vi "apply control changes.vi"(9 "new":string[][](array[string]), 10 "old":string[][](array[string]), 11 "Data In":T1[](array[typedef])) -> (1 "Changed indices":i32[](array[numeric]), 3 "Data Out":T1[](array[typedef]))   [LabVIEW 2016, in "update vi properties.lvlib"]
uses:
  update vi properties.lvlib
  Cluster_Data.ctl
  <vilib>/picture/picture.llb/imagedata.ctl
panel:
  # "Connector Pane"
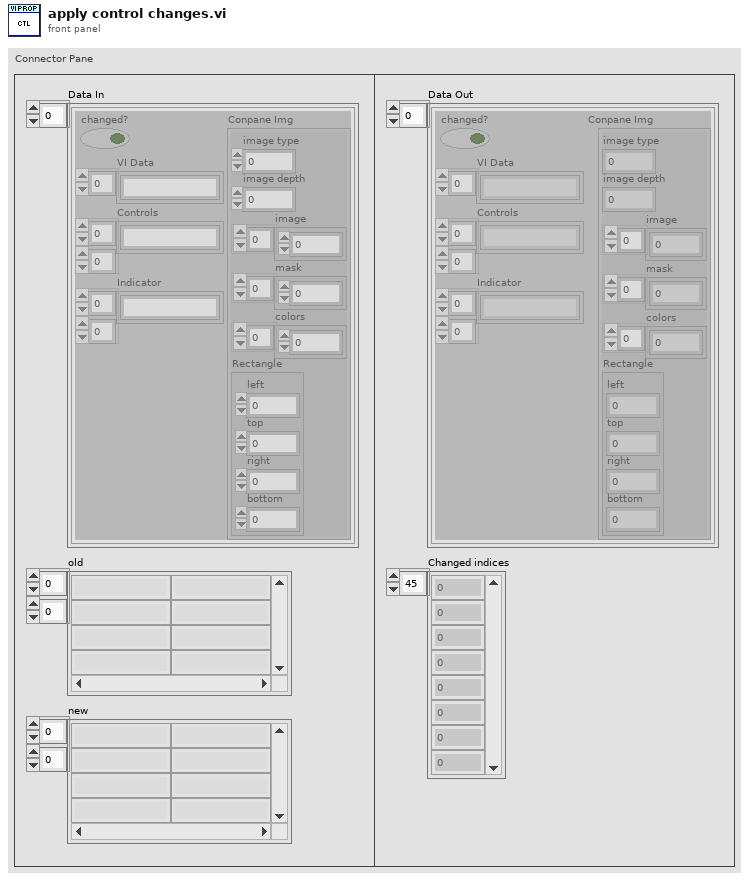
[diagram p1: front panel]
types:
  T1 = typedef "update vi properties.lvlib/Cluster_Data.ctl" = cluster{"changed?":bool, "VI Data":string[], "Controls":string[][], "Indicator":string[][], "Conpane Img":T2}
  T2 = typedef "imagedata.ctl" = cluster{"image type":i32, "image depth":i32, "image":u8[], "mask":u8[], "colors":u32[], "Rectangle":cluster{"left":i16, "top":i16, "right":i16, "bottom":i16}}
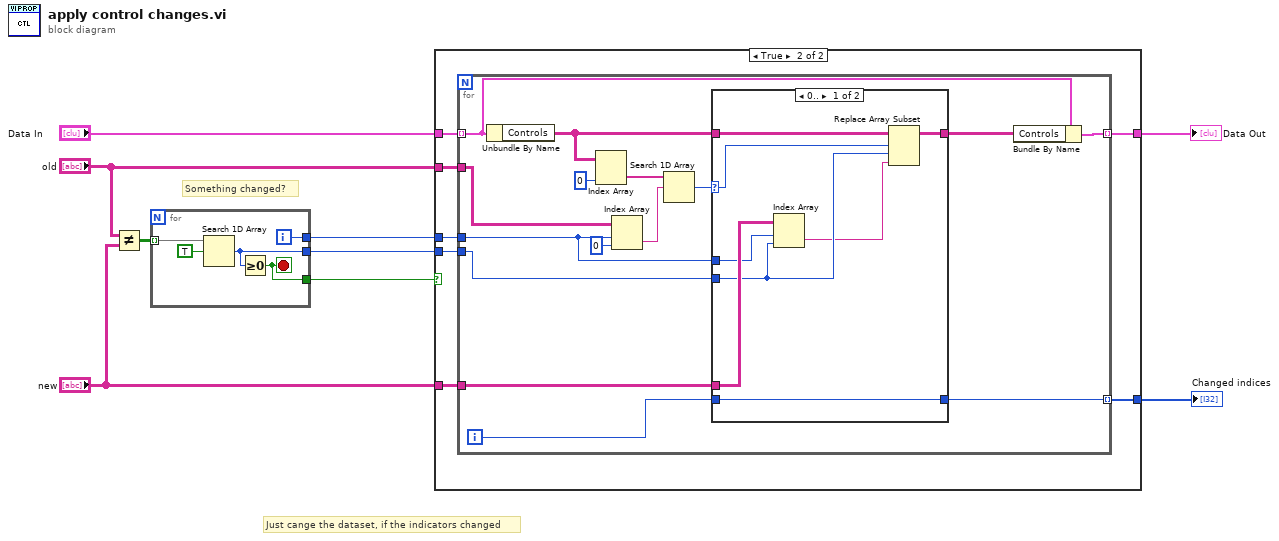
[diagram p0: block diagram]
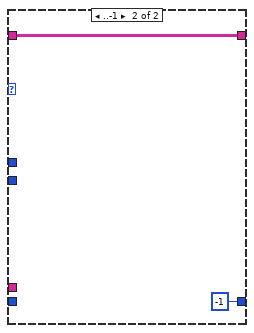
[diagram p3: hidden frame]
diagram:
  # "Just cange the dataset, if the indicators changed"
  # "Something changed?"
  n1 = Not Equal?(x="old", y="new") -> (x != y?=w9:bool[][])
  n2 = for {
    tunnel: w9 -> [w14] mode=indexing
    tunnel: [w12] -> w4
    tunnel: [w11] -> w5
    tunnel: [w10] -> w1
    i -> [w11]
    stop <- w10 stop-if-true
    n3 = Search 1D Array(1D array=w14, element=TRUE) -> (index of element=w12:i32)  [unwired: 1 in]
    n4 = Greater Or Equal To 0?(x=w12) -> (x >= 0?=w10:bool)
  }
  n5 = case shown="True" w1 {
    tunnel: "Data In" -> [w15 w22]
    tunnel: [w15 w18] -> w7
    tunnel: "old" -> [_ w21]
    tunnel: w5 -> [_ w20]
    tunnel: w4 -> [_ w19]
    tunnel: "new" -> [_ w17]
    tunnel: [_ w16] -> w2
    frame False {
    }
    frame True {
      n6 = for {
        tunnel: w22 -> [w25] mode=indexing
        tunnel: w21 -> [w35]
        tunnel: w20 -> [w29]
        tunnel: w19 -> [w31]
        tunnel: [w23] -> w18 mode=indexing
        tunnel: w17 -> [w30]
        tunnel: [w28] -> w16 mode=indexing
        i -> [w27]
        n7 = Unbundle By Name(w25) -> ("Controls"=w26:string[][])
        n8 = Index Array(array=w26, index (col)=0 ("disabled index (col)")) -> (element=w34:string[])  [unwired: 1 in]
        n9 = Index Array(array=w35, index (row)=w29, index (col)=0 ("disabled index (col)")) -> (element=w33:string)
        n10 = Search 1D Array(1D array=w34, element=w33) -> (index of element=w32:i32)  [unwired: 1 in]
        n11 = case shown="0.." w32 {
          selector: w32 -> [w39 _]
          tunnel: w26 -> [w45 w47]
          tunnel: [w44 w47] -> w24
          tunnel: w31 -> [w41 _]
          tunnel: w30 -> [w43 _]
          tunnel: w29 -> [w42 _]
          tunnel: [w38 -1 ("index of element")] -> w28
          tunnel: w27 -> [w38 _]
          frame 0.. {
            n12 = Index Array(array=w43, index (row)=w42, index (col)=w41) -> (element=w40:string)
            n13 = Replace Array Subset(array=w45, new element=w40, index (row)=w39, index (col)=w41) -> (w44:string[][])
          }
          frame ..-1 {
          }
        }
        n14 = Bundle By Name(cluster=w25, "Controls"=w24) -> (w23:T1)
      }
    }
  }
  "Data Out" <- w7
  "Changed indices" <- w2
